vi "SetSize.vi"(8 "error in (no error)":errorcluster, 10 "Size":u32, 11 "MultiBandState in":refnum<class "MultiBandState.lvclass">) -> (0 "error out":errorcluster, 3 "MultiBandState out":refnum<class "MultiBandState.lvclass">)   [LabVIEW 2018, in "Functions.lvlib" / "MultiBandState.lvclass"]
uses:
  MultiBandState.lvclass
  MultiBandState.lvclass/MultiBandState.ctl
  Accessors/Read MultiBand.vi
  Accessors/Write MultiBand.vi
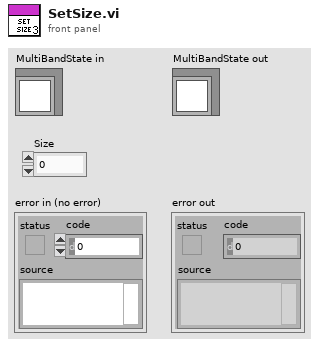
[diagram p1: front panel]
types:
  T1 = typedef "NI_Matrix.lvlib/RealMatrix.ctl" = dbl[][]
  T2 = cluster{"Handle":string, "Size":i32, "Gain":dbl, "Offset":dbl, "A":T1, "B":T1, "C":T1, "D":T1, "X":T1, "Waveform":waveform(dbl)}[]
  T3 = cluster{"Handle":string, "Size":i32, "Gain":dbl, "Offset":dbl, "A":T1, "B":T1, "C":T1, "D":T1, "X":T1, "Waveform":waveform(dbl)}
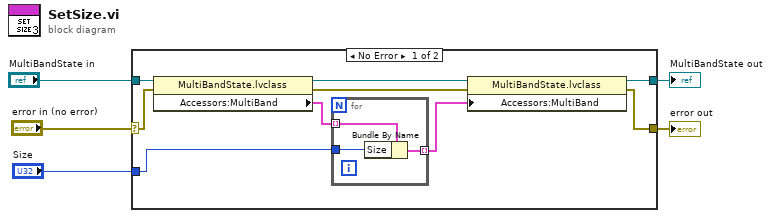
[diagram p0: block diagram]
diagram:
  n1 = case shown="No Error" "error in (no error)" {
    selector: "error in (no error)" -> [w7 w19]
    tunnel: [w12 w19] -> w4
    tunnel: "MultiBandState in" -> [w14 w18]
    tunnel: [w13 w18] -> w2
    tunnel: "Size" -> [w8 _]
    frame No Error {
      n2 = property class="MultiBandState.lvclass"(reference=w14, error in=w7) -> (reference out=w10:refnum<class "MultiBandState.lvclass">, error out=w9:errorcluster, "Accessors:MultiBand"=w11:T2)
      n3 = for {
        tunnel: w11 -> [w17] mode=indexing
        tunnel: w8 -> [w16]
        tunnel: [w15] -> w6 mode=indexing
        n4 = Bundle By Name(cluster=w17, "Size"=w16) -> (w15:T3)
      }
      n5 = property class="MultiBandState.lvclass"(reference=w10, error in=w9, "Accessors:MultiBand"=w6) -> (reference out=w13:refnum<class "MultiBandState.lvclass">, error out=w12:errorcluster)
    }
    frame Error {
    }
  }
  "error out" <- w4
  "MultiBandState out" <- w2
